vi "Get Node Class.vi"(8 "error in (no error)":errorcluster, 10 "Node Name":string, 11 "CI Deserializer in":refnum<class "CI Deserializer.lvclass">) -> (0 "error out":errorcluster, 2 "Node Class":string, 3 "CI Deserializer out":refnum<class "CI Deserializer.lvclass">)   [LabVIEW 2014, in "CI Deserializer.lvclass"]
uses:
  CI Deserializer.lvclass
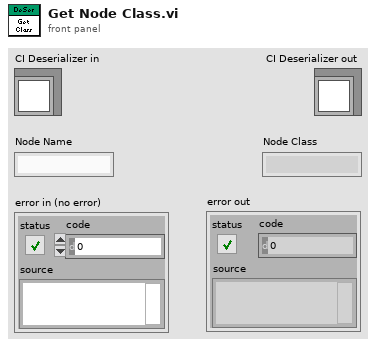
[diagram p1: front panel]
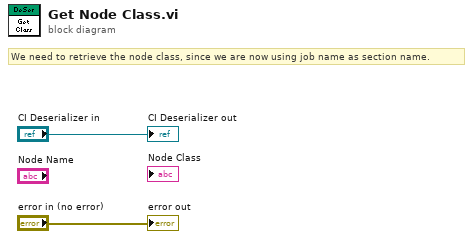
[diagram p0: block diagram]
diagram:
  # "We need to retrieve the node class, since we are now using job name as section name."
  "CI Deserializer out" <- "CI Deserializer in"
  "error out" <- "error in (no error)"
